vi "GUI Interlock Tester.vi"(8 "error in (no error)":errorcluster) -> (0 "error out":errorcluster)   [LabVIEW 2018]
uses:
  GUI Interlock Tester-case.ctl
  <vilib>/addons/_JKI Toolkits/Caraya/classes/Test/Test.lvclass
  <vilib>/addons/_JKI Toolkits/Caraya/classes/Assert/Assert.lvclass
  Libraries/Device Under Test_Cloneable_DQMH/Device Under Test_Cloneable_DQMH.lvlib
panel:
  in  "Self Test Button":bool
  in  "Power Off Button":bool
  in  "Power On Button":bool
  # "The buttons below are not intended to be inputs. Their only role is to be \nused inside this VI for the tests."
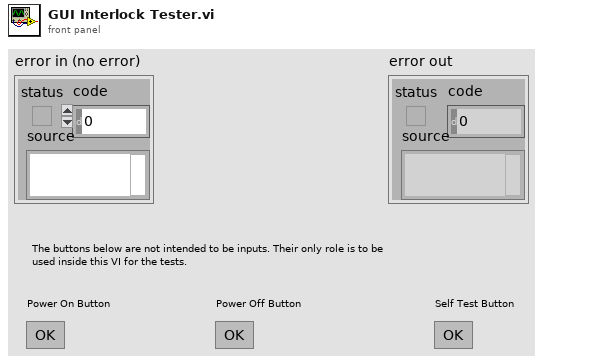
[diagram p1: front panel]
types:
  T1 = typedef "GUI Interlock Tester-case.ctl" = cluster{"test case ID":string, "Expected Power On Button Disabled":enum8{"Enabled", "Disabled", "Disabled and Grayed Out"}, "Expected Power Off Button Disabled":enum8{"Enabled", "Disabled", "Disabled and Grayed Out"}, "Expected Self Test Button Disabled":enum8{"Enabled", "Disabled", "Disabled and Grayed Out"}, "Power State":bool}
  T2 = enum8{"Enabled", "Disabled", "Disabled and Grayed Out"}
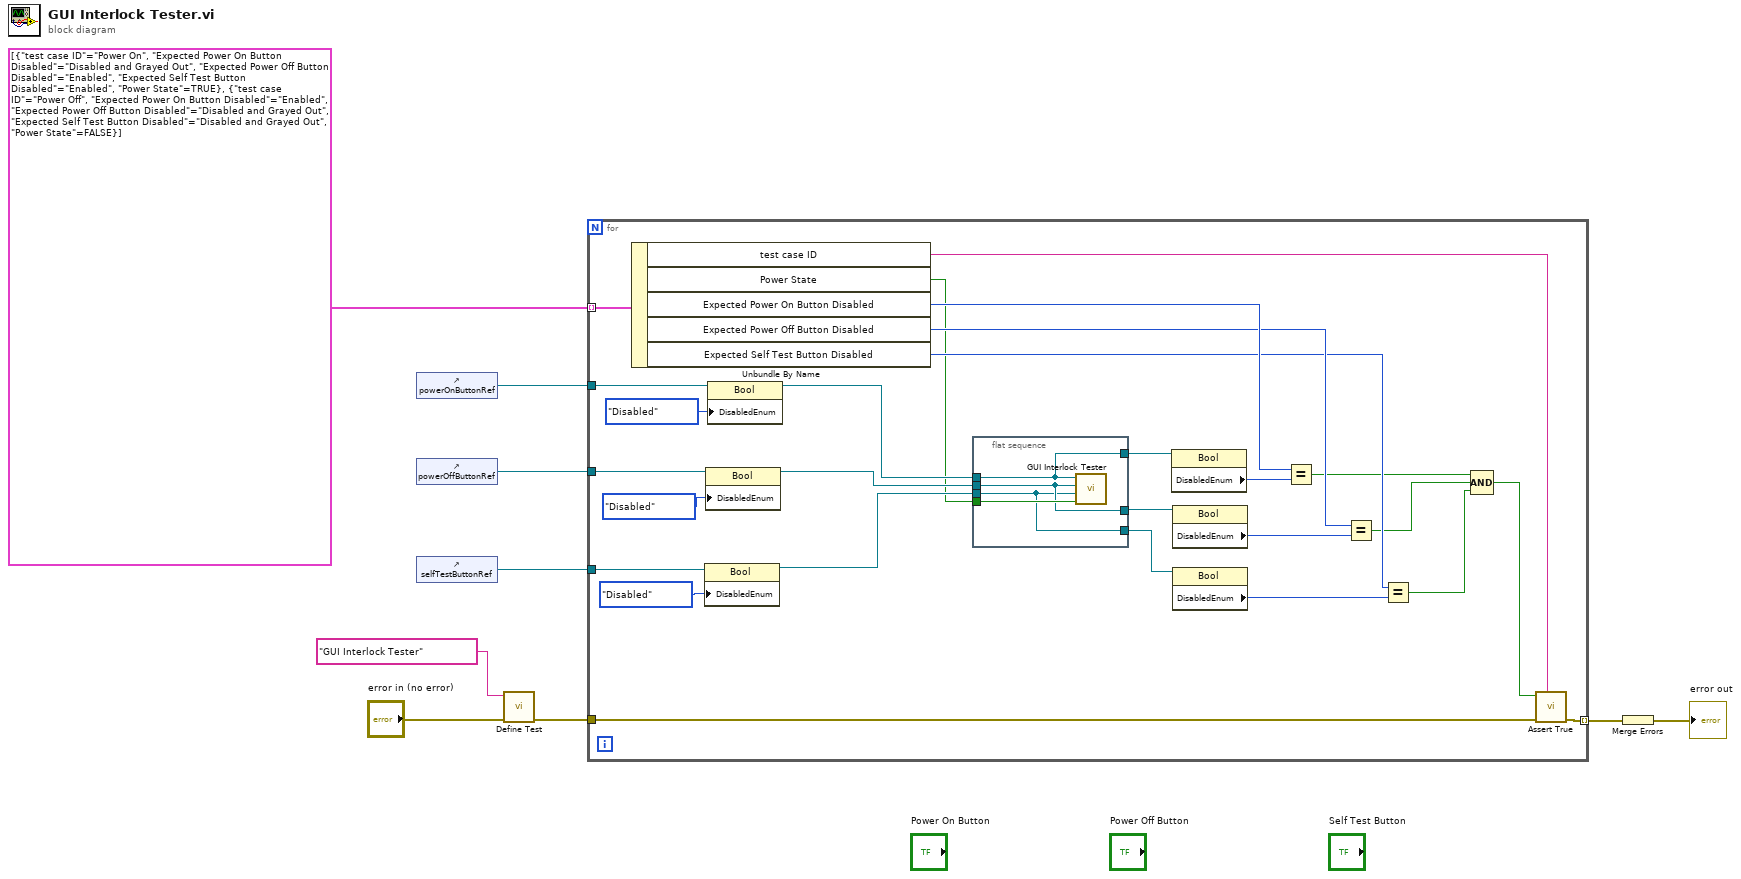
[diagram p0: block diagram]
diagram:
  n1 = control-ref of="powerOnButtonRef"() -> (w8:refnum<vi>)
  n2 = control-ref of="powerOffButtonRef"() -> (w7:refnum<vi>)
  n3 = control-ref of="selfTestButtonRef"() -> (w6:refnum<vi>)
  n4 = call <vilib>:"Define Test.vi"("error in (no error)"="error in (no error)", "Label (VI Title)"="GUI Interlock Tester") -> ("error out"=w2:errorcluster)  [unwired: 9 in]
  n5 = for {
    tunnel: w8 -> [w33]
    tunnel: w7 -> [w32]
    tunnel: w6 -> [w31]
    tunnel: T1[] [{"test case ID"="Power On", "Expected Power On Button Disabled"=enum."Disabled and Grayed Out", "Expected Power Off Button Disabled"=enum."Enabled", "Expected Self Test Button Disabled"=enum."Enabled", "Power State"=TRUE}, {"test case ID"="Power Off", "Expected Power On Button Disabled"=enum."Enabled", "Expected Power Off Button Disabled"=enum."Disabled and Grayed Out", "Expected Self Test Button Disabled"=enum."Disabled and Grayed Out", "Power State"=FALSE}] -> [w30] mode=indexing
    tunnel: [w13] -> w3 mode=indexing
    tunnel: w2 -> [w12]
    n6 = Unbundle By Name(w30) -> ("test case ID"=w11:string, "Power State"=w10:bool, "Expected Power On Button Disabled"=w23:T2, "Expected Power Off Button Disabled"=w20:T2, "Expected Self Test Button Disabled"=w18:T2)
    n7 = property class="Bool"(reference=w31, "DisabledEnum"=T2."Disabled" ("Disabled")) -> (reference out=w27:refnum<vi>)  [unwired: 1 in, 1 out]
    n8 = property class="Bool"(reference=w32, "DisabledEnum"=T2."Disabled" ("Disabled")) -> (reference out=w28:refnum<vi>)  [unwired: 1 in, 1 out]
    n9 = property class="Bool"(reference=w33, "DisabledEnum"=T2."Disabled" ("Disabled")) -> (reference out=w29:refnum<vi>)  [unwired: 1 in, 1 out]
    n10 = flat-sequence {
      tunnel: w10 -> [w40]
      tunnel: w29 -> [w39]
      tunnel: w28 -> [w38]
      tunnel: w27 -> [w37]
      tunnel: [w39] -> w26
      tunnel: [w38] -> w25
      tunnel: [w37] -> w24
      frame #0 {
        n11 = call "GUI Interlock Tester.vi"("Power State"=w40, "Self Test Button"=w37, "Power Off Button"=w38, "Power On Button"=w39) -> ()  [unwired: 8 in]
      }
    }
    n12 = property class="Bool"(reference=w26) -> ("DisabledEnum"=w22:T2)  [unwired: 1 in, 2 out]
    n13 = property class="Bool"(reference=w25) -> ("DisabledEnum"=w21:T2)  [unwired: 1 in, 2 out]
    n14 = property class="Bool"(reference=w24) -> ("DisabledEnum"=w19:T2)  [unwired: 1 in, 2 out]
    n15 = Equal?(x=w23, y=w22) -> (x = y?=w17:bool)
    n16 = Equal?(x=w20, y=w21) -> (x = y?=w16:bool)
    n17 = Equal?(x=w18, y=w19) -> (x = y?=w15:bool)
    n18 = Compound Arithmetic op=AND(w17, w16, w15) -> (w14:bool)
    n19 = call <vilib>:"Assert True.vi"("Label"=w11, "error in (no error)"=w12, "True?"=w14) -> ("error out"=w13:errorcluster)  [unwired: 8 in]
  }
  n20 = Merge Errors(w3) -> (→"error out":errorcluster)
